vi "Prepare Config Files.vi"(8 "error in":errorcluster, 11 "Project Root":path) -> (0 "error out":errorcluster, 3 "Config Directory":path)   [LabVIEW 2011]
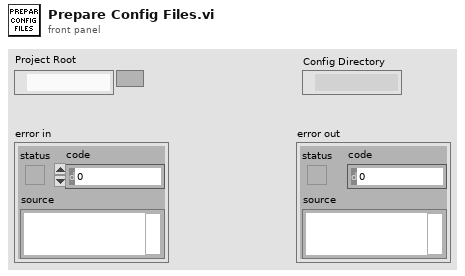
[diagram p1: front panel]
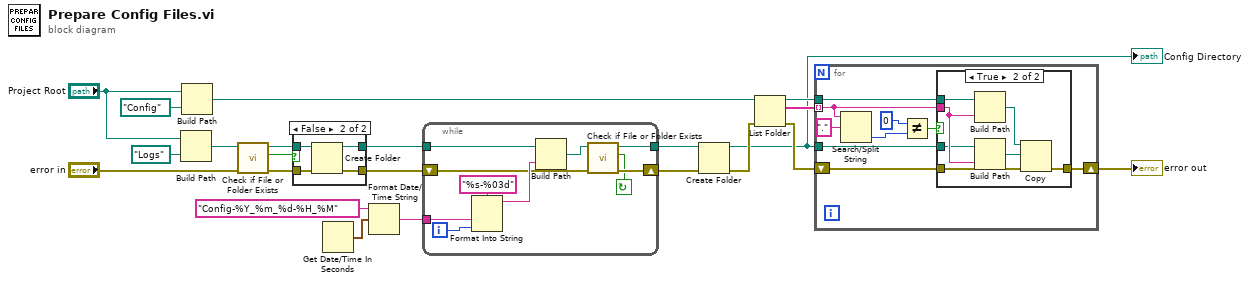
[diagram p0: block diagram]
diagram:
  n1 = Build Path(base path="Project Root", name or relative path=path "Logs") -> (appended path=w19:path)
  n2 = Build Path(base path="Project Root", name or relative path=path "Config") -> (appended path=w2:path)
  n3 = call <vilib>:"Check if File or Folder Exists.vi"("error in (no error)"="error in", "path"=w19) -> ("error out"=w17:errorcluster, "file or folder exists?"=w15:bool, "dup path"=w16:path)  [unwired: 7 in]
  n4 = case shown="False" w15 {
    tunnel: [w24 w28] -> w13
    tunnel: [w23 w27] -> w14
    tunnel: w17 -> [w23 w26]
    tunnel: w16 -> [w24 w25]
    frame True {
    }
    frame False {
      n5 = Create Folder(path (use dialog)=w25, error in=w26) -> (created path=w28:path, error out=w27:errorcluster)  [unwired: 1 in, 1 out]
    }
  }
  n6 = Get Date/Time In Seconds() -> (seconds since 1Jan1904=w21:timestamp)
  n7 = Format Date/Time String(time format string (%c)="Config-%Y_%m_%d-%H_%M", seconds (now)=w21) -> (date/time string=w12:string)  [unwired: 1 in]
  n8 = while {
    tunnel: w13 -> [w35]
    tunnel: w12 -> [w36]
    shift-right: [w31] -> w11
    shift-left: w14 -> [w32]
    tunnel: [w29] -> w10
    i -> [w37]
    stop <- w30 continue-if-true
    n9 = Format Into String(format string="%s-%03d", w36, w37) -> (resulting string=w34:string)  [unwired: 2 in, 1 out]
    n10 = Build Path(base path=w35, name or relative path=w34) -> (appended path=w33:path)
    n11 = call <vilib>:"Check if File or Folder Exists.vi"("error in (no error)"=w32, "path"=w33) -> ("error out"=w31:errorcluster, "file or folder exists?"=w30:bool, "dup path"=w29:path)  [unwired: 7 in]
  }
  n12 = Create Folder(path (use dialog)=w10, error in=w11) -> (created path=w1:path, error out=w9:errorcluster)  [unwired: 1 in, 1 out]
  "Config Directory" <- w1
  n13 = List Folder(path=w2, error in=w9) -> (path out=w7:path, filenames=w8:string[], error out=w6:errorcluster)  [unwired: 2 in, 1 out]
  n14 = for {
    tunnel: w8 -> [w43] mode=indexing
    tunnel: w7 -> [w47]
    tunnel: w1 -> [w44]
    shift-right: [w45] -> w5
    shift-left: w6 -> [w46]
    n15 = Search/Split String(string=w43, search string/char (-)=".") -> (offset of match=w40:i32)  [unwired: 1 in, 2 out]
    n16 = Not Equal?(x=0, y=w40) -> (x != y?=w41:bool)
    n17 = case shown="True" w41 {
      tunnel: w47 -> [_ w55]
      tunnel: w43 -> [_ w54]
      tunnel: w46 -> [w48 w53]
      tunnel: [w48 w50] -> w45
      tunnel: w44 -> [_ w49]
      frame False {
      }
      frame True {
        n18 = Build Path(base path=w55, name or relative path=w54) -> (appended path=w52:path)
        n19 = Build Path(base path=w49, name or relative path=w54) -> (appended path=w51:path)
        n20 = Copy(8:w53, 10:w51, 11:w52) -> (0:w50:errorcluster)  [unwired: 2 in, 2 out]
      }
    }
  }
  "error out" <- w5
